vi "Run Controller.vi"(8 "Error In":errorcluster, 9 "Run Selector":bool=TRUE, 10 "Interlock Check Output":string, 11 "Cluster Data In":T1) -> (0 "Error Out":errorcluster, 3 "Cluster Data Out":T1)   [LabVIEW 2024]
uses:
  Controls/Data Cluster.ctl
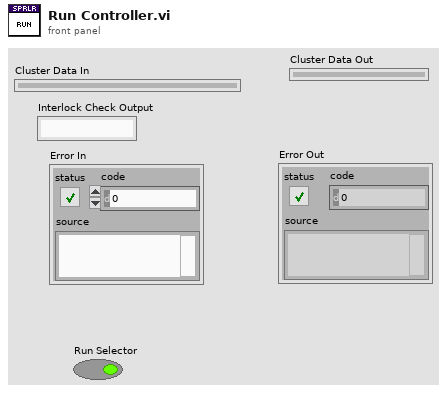
[diagram p1: front panel]
types:
  T1 = typedef "Data Cluster.ctl" = cluster{"Zone Setup Array Actual":cluster{"Zone Selector":string, "Timing":dbl}[], "Zone Setup Array Current":cluster{"Zone Selector":string, "Timing":dbl}[], "Zone Indicators":cluster{"North":bool, "East":bool, "South":bool, "West":bool, "Timing":u32}, "Controller Status":string, "Water Pressure Sensor (%)":u32, "Rain Sensor":bool, "Current Zone Active?":bool, "Time Elapsed?":bool, "QueueRefOut":refnum<queue>}
  T2 = enum16{"Create", "Enqueue", "Dequeue", "Enstack", "Flush", "Release"}
  T3 = cluster{"North":bool, "East":bool, "South":bool, "West":bool, "Timing":u32}
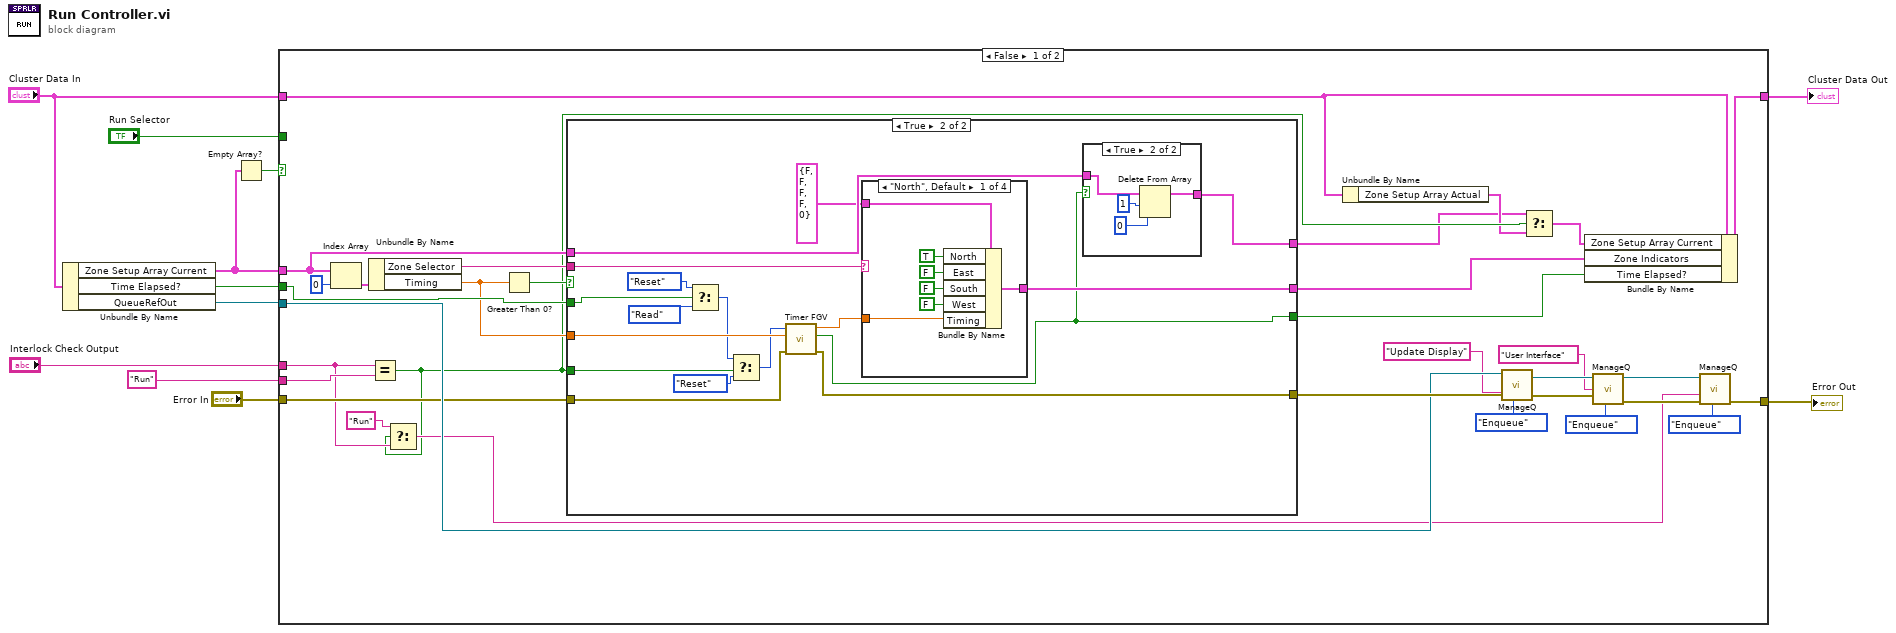
[diagram p0: block diagram]
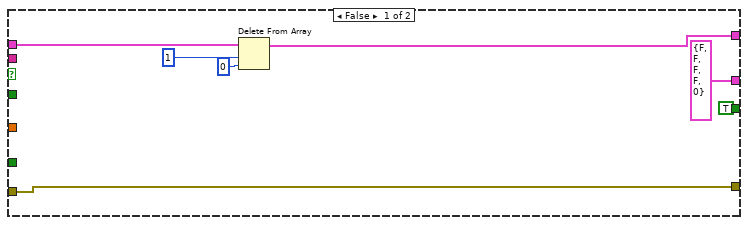
[diagram p2: hidden frame]
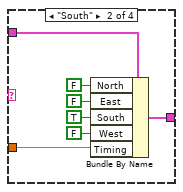
[diagram p4: hidden frame]
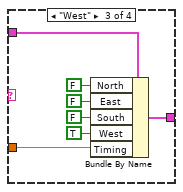
[diagram p5: hidden frame]
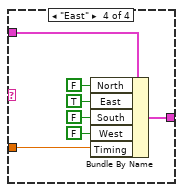
[diagram p6: hidden frame]
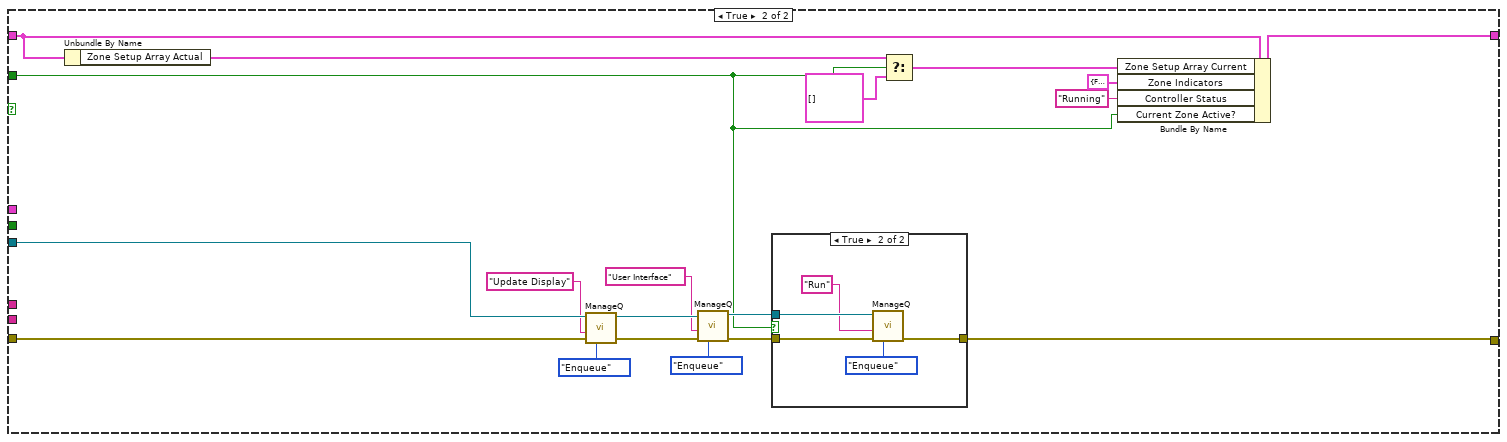
[diagram p7: hidden frame]
diagram:
  n1 = Unbundle By Name("Cluster Data In") -> ("Zone Setup Array Current"=w7:cluster{"Zone Selector":string, "Timing":dbl}[], "Time Elapsed?"=w11:bool, "QueueRefOut"=w9:refnum<queue>)
  n2 = Empty Array?(array=w7) -> (empty?=w6:bool)
  n3 = case shown="False" w6 {
    tunnel: w11 -> [w40 _]
    tunnel: w7 -> [w35 _]
    tunnel: "Run" ("y") -> [w34 _]
    tunnel: w9 -> [w32 w107]
    tunnel: "Interlock Check Output" -> [w18 _]
    tunnel: "Run Selector" -> [_ w101]
    tunnel: "Cluster Data In" -> [w16 w119]
    tunnel: [w20 w115] -> w3
    tunnel: "Error In" -> [w22 w111]
    tunnel: [w21 w102] -> w1
    frame False {
      n4 = Index Array(array=w35, index=0) -> (element=w42:cluster{"Zone Selector":string, "Timing":dbl})
      n5 = Unbundle By Name(w42) -> ("Zone Selector"=w41:string, "Timing"=w39:dbl)
      n6 = Equal?(x=w18, y=w34) -> (x = y?=w15:bool)
      n7 = Select(t="Run" ("State In"), s=w15, f=w18) -> (s? t:f=w17:string)
      n8 = Greater Than 0?(x=w39) -> (x > 0?=w38:bool)
      n9 = case shown="True" w38 {
        tunnel: w41 -> [_ w67]
        tunnel: w39 -> [_ w66]
        tunnel: w40 -> [_ w54]
        tunnel: w15 -> [_ w55]
        tunnel: [T3 {"North"=FALSE, "East"=FALSE, "South"=FALSE, "West"=FALSE, "Timing"=0} ("Zone Indicators") w65] -> w36
        tunnel: [TRUE ("Time Elapsed?") w64] -> w37
        tunnel: w35 -> [w48 w62]
        tunnel: [w45 w63] -> w12
        tunnel: w22 -> [w44 w61]
        tunnel: [w44 w60] -> w33
        frame False {
          n10 = Delete From Array(array=w48, length=1, index=0) -> (array with subset deleted=w45:cluster{"Zone Selector":string, "Timing":dbl}[])  [unwired: 1 out]
        }
        frame True {
          n11 = Select(t=enum16{"Reset", "Read", "Pause"}."Reset" ("Timer state"), s=w54, f=enum16{"Reset", "Read", "Pause"}."Read" ("Timer state")) -> (s? t:f=w51:enum16{"Reset", "Read", "Pause"})
          n12 = Select(t=w51, s=w55, f=enum16{"Reset", "Read", "Pause"}."Reset" ("Timer state")) -> (s? t:f=w53:enum16{"Reset", "Read", "Pause"})
          n13 = call "Timer FGV.vi"("Error In"=w61, "Time Target (s)"=w66, "Timer state"=w53) -> ("Error Out"=w60:errorcluster, "Time Elapsed?"=w64:bool, "Elapsed Time"=w56:dbl)  [unwired: 6 in]
          n14 = case shown="\"North\", Default" w67 {
            tunnel: T3 {"North"=FALSE, "East"=FALSE, "South"=FALSE, "West"=FALSE, "Timing"=0} ("Zone Indicators") -> [w79 w86 w93 w100]
            tunnel: w56 -> [w78 w85 w92 w99]
            tunnel: [w73 w80 w87 w94] -> w65
            frame "North", Default {
              n15 = Bundle By Name(cluster=w79, "North"=TRUE, "East"=FALSE, "South"=FALSE, "West"=FALSE, "Timing"=w78) -> (w73:T3)
            }
            frame "South" {
              n16 = Bundle By Name(cluster=w86, "North"=FALSE, "East"=FALSE, "South"=TRUE, "West"=FALSE, "Timing"=w85) -> (w80:T3)
            }
            frame "West" {
              n17 = Bundle By Name(cluster=w93, "North"=FALSE, "East"=FALSE, "South"=FALSE, "West"=TRUE, "Timing"=w92) -> (w87:T3)
            }
            frame "East" {
              n18 = Bundle By Name(cluster=w100, "North"=FALSE, "East"=TRUE, "South"=FALSE, "West"=FALSE, "Timing"=w99) -> (w94:T3)
            }
          }
          n19 = case shown="True" w64 {
            tunnel: w62 -> [w68 w72]
            tunnel: [w68 w69] -> w63
            frame False {
            }
            frame True {
              n20 = Delete From Array(array=w72, length=1, index=0) -> (array with subset deleted=w69:cluster{"Zone Selector":string, "Timing":dbl}[])  [unwired: 1 out]
            }
          }
        }
      }
      n21 = Unbundle By Name(w16) -> ("Zone Setup Array Actual"=w14:cluster{"Zone Selector":string, "Timing":dbl}[])
      n22 = call "ManageQ.vi"("QStateIn"=T2."Enqueue", "Error In"=w33, "State In"="Update Display", "QueueRefIn"=w32) -> ("Error Out"=w30:errorcluster, "QueueRefOut"=w28:refnum<queue>)  [unwired: 5 in, 1 out]
      n23 = Select(t=w12, s=w15, f=w14) -> (s? t:f=w13:cluster{"Zone Selector":string, "Timing":dbl}[])
      n24 = Bundle By Name(cluster=w16, "Zone Setup Array Current"=w13, "Zone Indicators"=w36, "Time Elapsed?"=w37) -> (w20:T1)
      n25 = call "ManageQ.vi"("QStateIn"=T2."Enqueue", "Error In"=w30, "State In"="User Interface", "QueueRefIn"=w28) -> ("Error Out"=w29:errorcluster, "QueueRefOut"=w26:refnum<queue>)  [unwired: 5 in, 1 out]
      n26 = call "ManageQ.vi"("QStateIn"=T2."Enqueue", "Error In"=w29, "State In"=w17, "QueueRefIn"=w26) -> ("Error Out"=w21:errorcluster)  [unwired: 5 in, 2 out]
    }
    frame True {
      n27 = Unbundle By Name(w119) -> ("Zone Setup Array Actual"=w118:cluster{"Zone Selector":string, "Timing":dbl}[])
      n28 = call "ManageQ.vi"("QStateIn"=T2."Enqueue", "Error In"=w111, "State In"="Update Display", "QueueRefIn"=w107) -> ("Error Out"=w109:errorcluster, "QueueRefOut"=w106:refnum<queue>)  [unwired: 5 in, 1 out]
      n29 = call "ManageQ.vi"("QStateIn"=T2."Enqueue", "Error In"=w109, "State In"="User Interface", "QueueRefIn"=w106) -> ("Error Out"=w108:errorcluster, "QueueRefOut"=w105:refnum<queue>)  [unwired: 5 in, 1 out]
      n30 = case shown="True" w101 {
        tunnel: w108 -> [w120 w124]
        tunnel: w105 -> [_ w123]
        tunnel: [w120 w121] -> w102
        frame False {
        }
        frame True {
          n31 = call "ManageQ.vi"("QStateIn"=T2."Enqueue", "Error In"=w124, "State In"="Run", "QueueRefIn"=w123) -> ("Error Out"=w121:errorcluster)  [unwired: 5 in, 2 out]
        }
      }
      n32 = Select(t=w118, s=w101, f=cluster{"Zone Selector":string, "Timing":dbl}[] []) -> (s? t:f=w116:cluster{"Zone Selector":string, "Timing":dbl}[])
      n33 = Bundle By Name(cluster=w119, "Zone Setup Array Current"=w116, "Zone Indicators"=T3 {"North"=FALSE, "East"=FALSE, "South"=FALSE, "West"=FALSE, "Timing"=0}, "Controller Status"="Running", "Current Zone Active?"=w101) -> (w115:T1)
    }
  }
  "Cluster Data Out" <- w3
  "Error Out" <- w1
